vi "3-9.vi"() -> ()   [LabVIEW 2014]
panel:
  out "Wind 2":string
  in  "Max Wind Speed":dbl
  in  "Wind Speed":dbl
  in  "Current temp 2":dbl
  out "Boolean":bool
  out "Temp":string
  in  "minimum temp":dbl
  in  "max temp":dbl
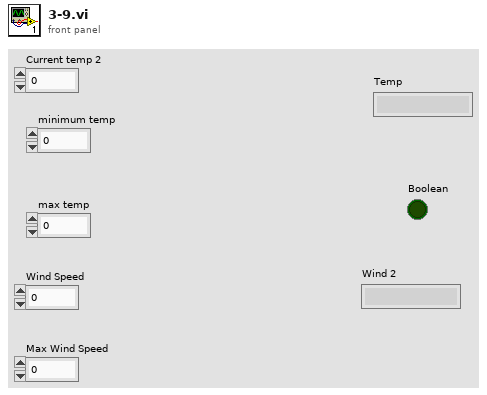
[diagram p1: front panel]
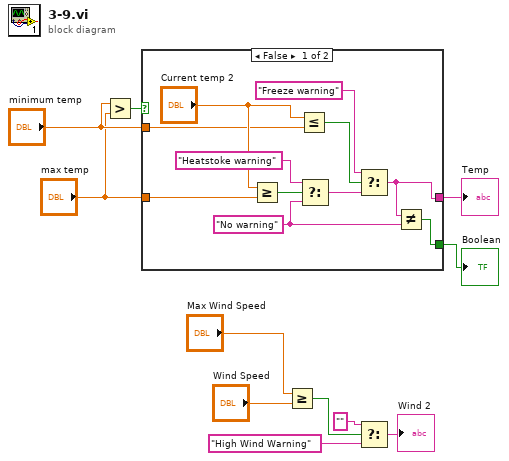
[diagram p0: block diagram]
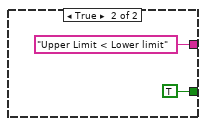
[diagram p2: hidden frame]
diagram:
  n1 = Greater?(x="minimum temp", y="max temp") -> (0:w9:bool)
  n2 = case shown="False" w9 {
    tunnel: [w14 "Upper Limit < Lower limit"] -> w11
    tunnel: [w15 TRUE] -> w10
    tunnel: "minimum temp" -> [w13 _]
    tunnel: "max temp" -> [w12 _]
    frame False {
      w17 = "No warning"
      n3 = Greater Or Equal?(x="Current temp 2", y=w12) -> (x >= y?=w22:bool)
      n4 = Less Or Equal?(x="Current temp 2", y=w13) -> (x <= y?=w21:bool)
      n5 = Select(t="Heatstoke warning", s=w22, f=w17) -> (s? t:f=w18:string)
      n6 = Select(t="Freeze warning", s=w21, f=w18) -> (s? t:f=w14:string)
      n7 = Not Equal?(x=w14, y=w17) -> (x != y?=w15:bool)
    }
    frame True {
    }
  }
  "Temp" <- w11
  "Boolean" <- w10
  n8 = Greater Or Equal?(x="Max Wind Speed", y="Wind Speed") -> (x >= y?=w4:bool)
  n9 = Select(t="", s=w4, f="High Wind Warning") -> (s? t:f=→"Wind 2":string)
